vi "Clear DTCs Event.vi"(0 "connection info":T1, 1 "Addresses":refnum<vi>, 5 "State Variables":T3, 7 "Address Lookup Table":variant, 12 "Error Q":refnum<queue>, 13 "VI Ref":refnum<vi>) -> (4 "connection info":T1, 8 "Address Lookup Table Out":variant)   [LabVIEW 2019, in "J1939 Workspace Shared.lvlib"]
uses:
  J1939 Workspace Shared.lvlib
  Addon/Addon Shared/J1939 Addon Shared.lvlib
  Types/Private Data.ctl
  Addon/Addon Shared/Types/Error Types.ctl
  Addon/Addon Shared/Types/Error Cluster.ctl
  <vilib>/NI/STM/SubVIs/MetaDataElement.ctl
  <vilib>/NI/STM/NI STM.lvlib
  <vilib>/NI/STM/TCP/TCP Connection Info.ctl
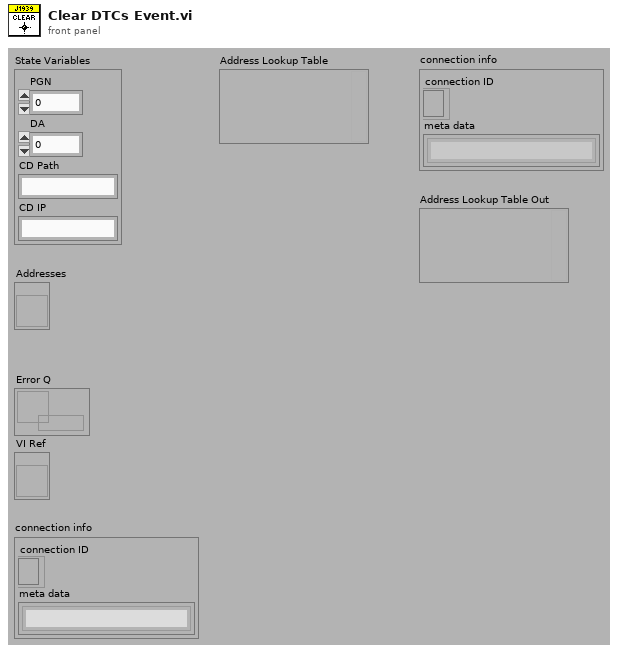
[diagram p1: front panel]
types:
  T1 = typedef "NI STM.lvlib/TCP Connection Info.ctl" = cluster{"connection ID":refnum<k5>, "meta data":T2[]}
  T2 = typedef "NI STM.lvlib/MetaDataElement.ctl" = string
  T3 = typedef "J1939 Workspace Shared.lvlib/Private Data.ctl" = cluster{"PGN":u32, "DA":u8, "CD Path":string, "CD IP":string}
  T4 = typedef "J1939 Workspace Shared.lvlib/Address Parse Tree Cluster.ctl" = cluster{"Parent Selection":string, "Address Selection":string, "CMD Selection":string}
  T5 = typedef "J1939 Addon Shared.lvlib/Error Cluster.ctl" = cluster{"error out":errorcluster, "Enum":T6, "Address":u8, "Timestamp":timestamp}
  T6 = typedef "J1939 Addon Shared.lvlib/Error Types.ctl" = enum16{"Request", "RAW Generation", "Clear Active DTCs", "Clear Previous DTCs", "Addresses", "TLAs", "Get Active DTCs", "Get Previous DTCs", "TCP Connection"}
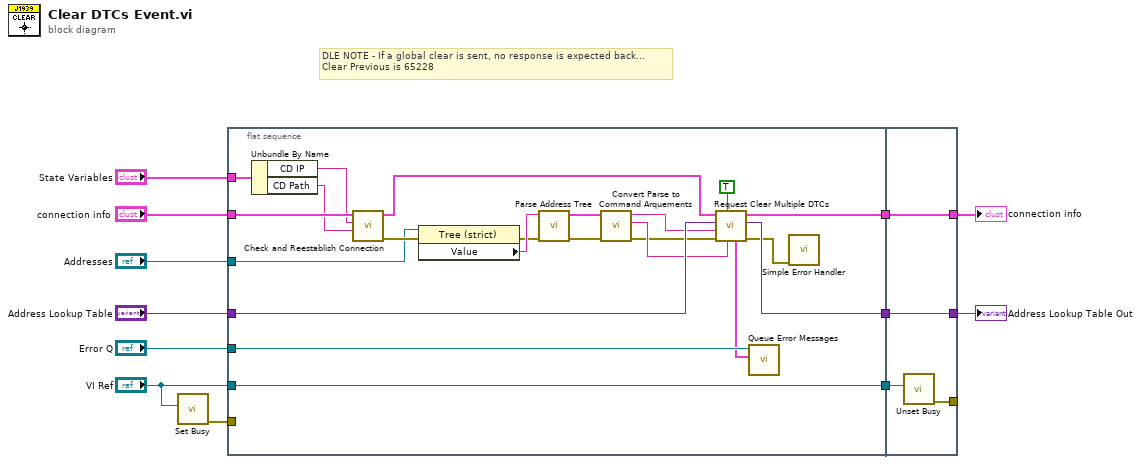
[diagram p0: block diagram]
diagram:
  # "DLE NOTE - If a global clear is sent, no response is expected back...\nClear Previous is 65228"
  n1 = call <vilib>:"Set Busy.vi"("VI reference (current VI)"="VI Ref") -> ("error out"=w6:errorcluster)  [unwired: 9 in, 1 out]
  n2 = flat-sequence {
    tunnel: "connection info" -> [w34]
    tunnel: "Address Lookup Table" -> [w29]
    tunnel: [w32] -> w12
    tunnel: [w28] -> w11
    tunnel: w6 -> [_]
    tunnel: "Error Q" -> [w21]
    tunnel: "State Variables" -> [w17]
    tunnel: [w14] -> w10
    tunnel: "VI Ref" -> [w14]
    tunnel: "Addresses" -> [w13]
    tunnel: [w37] -> w5
    tunnel: [w38] -> w3
    tunnel: w12 -> [w38]
    tunnel: w11 -> [w37]
    tunnel: [w36] -> _
    tunnel: w10 -> [w35]
    frame #0 {
      n3 = Unbundle By Name(w17) -> ("CD IP"=w15:string, "CD Path"=w16:string)
      n4 = call "Check and Reestablish Connection.vi"("CD Path"=w16, "IP Address"=w15, "connection info"=w34) -> ("error out"=w33:errorcluster, "connection info"=w24:T1)  [unwired: 7 in]
      n5 = property on="Property Node" class="Tree (strict)"(reference=w13, error in=w33) -> (error out=w25:errorcluster, "Value"=w31:string)  [unwired: 1 out]
      n6 = call "Parse Address Tree.vi"("error in"=w25, "Address Selection"=w31) -> ("error out"=w23:errorcluster, "Address Parsed Tree"=w30:T4)  [unwired: 8 in]
      n7 = call "Convert Parse to Command Arquements.vi"("error in (no error)"=w23, "Address Parsed Tree"=w30) -> ("error out"=w22:errorcluster, "Type"=w26:string, "Address"=w27:string)  [unwired: 7 in]
      n8 = call "Request Clear Multiple DTCs.vi"("Command"=w26, "Ignore Response"=TRUE, "error in"=w22, "Address"=w27, "Lookup Table"=w29, "connection info"=w24) -> ("error out"=w19:errorcluster, "Lookup Table"=w28:variant, "connection info"=w32:T1, "Error Array"=w20:T5[])  [unwired: 2 in]
      n9 = call "Queue Error Messages.vi"("Error Array"=w20, "queue out"=w21) -> ()  [unwired: 9 in, 1 out]
      n10 = call <vilib>:"Simple Error Handler.vi"("error in (no error)"=w19) -> ()  [unwired: 4 in, 5 out]
    }
    frame #1 {
      n11 = call <vilib>:"Unset Busy.vi"("VI reference (current VI)"=w35) -> ("error out"=w36:errorcluster)  [unwired: 10 in]
    }
  }
  "Address Lookup Table Out" <- w5
  "connection info" <- w3
